vi "test FPGA DIO.vi"(8 "error in (no error)":errorcluster, 11 "TestCase in":refnum<class "cRIO System Tests.lvclass">) -> (0 "error out":errorcluster, 3 "TestCase out":refnum<class "cRIO System Tests.lvclass">)   [LabVIEW 2020, in "cRIO System Tests.lvclass"]
uses:
  cRIO System Tests.lvclass
  C:/Program Files (x86)/National Instruments/LabVIEW 2020/vi.lib/NI/VeriStand Custom Device Testing Tools/VeriStandTestCase/VeriStandTestCase.lvclass
  <vilib>/numeric/Random Number (Range) U64.vi
  <vilib>/numeric/sub_Random U32.vi
  <vilib>/addons/_JKI Toolkits/VI Tester/TestCase.llb/TestCase.lvclass
  <vilib>/NI/VeriStand Custom Device Testing Tools/VeriStandTestCase/VeriStandTestCase.lvclass
  C:/Program Files (x86)/National Instruments/LabVIEW 2020/vi.lib/addons/_JKI Toolkits/VI Tester/TestCase.llb/TestCase.lvclass
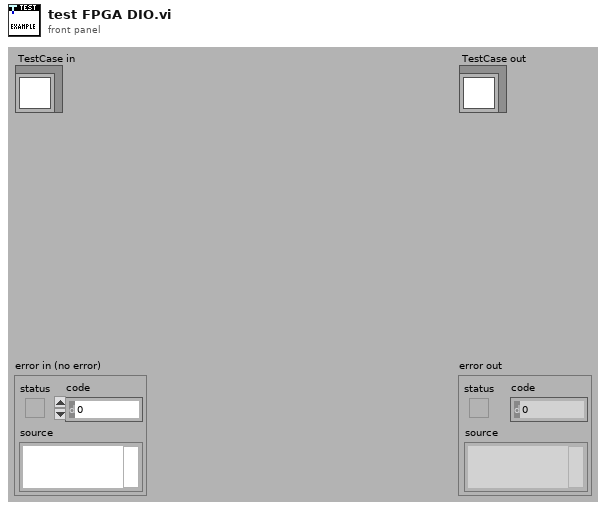
[diagram p1: front panel]
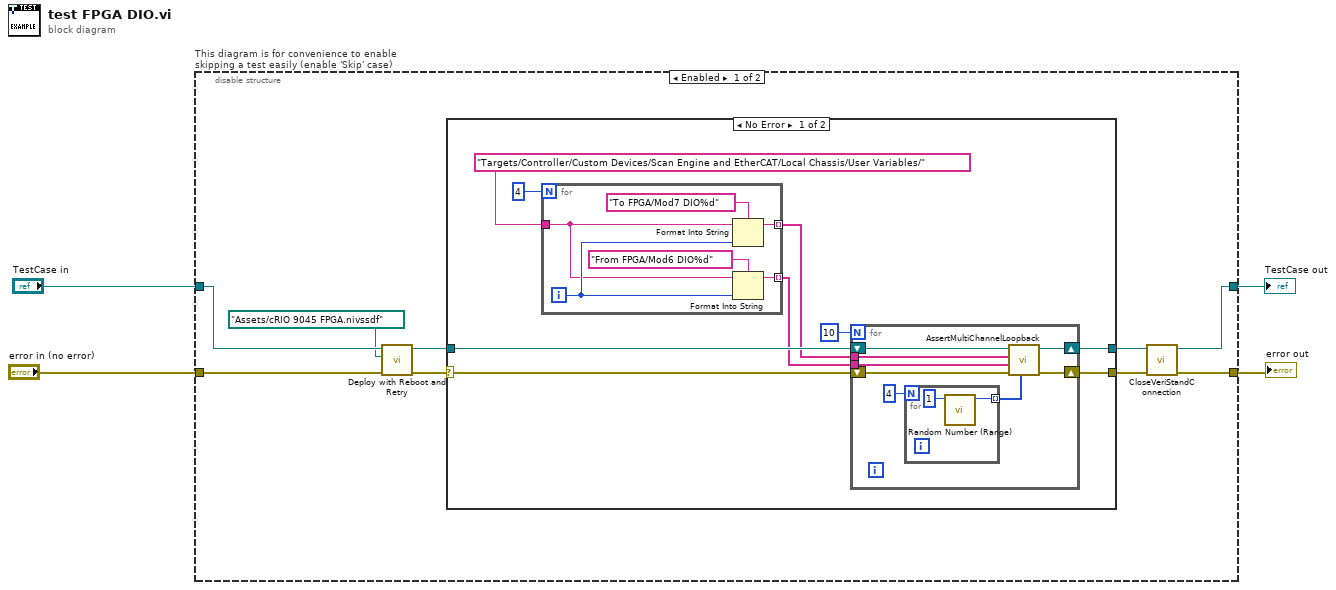
[diagram p0: block diagram]
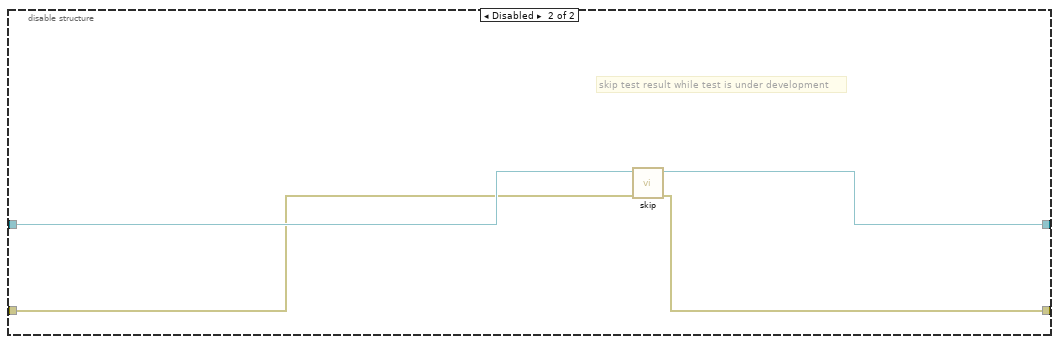
[diagram p3: hidden frame]
diagram:
  n1 = disable-structure "This diagram is for convenience to enable skipping a test easily (enable 'Skip' case)" shown="Enabled" {
    disable-tunnel: "TestCase in" -> [w10 w44]
    disable-tunnel: [w6 w42] -> w1
    disable-tunnel: [w8 w43] -> w3
    disable-tunnel: "error in (no error)" -> [w12 w41]
    frame Enabled {
      n2 = call "Deploy with Reboot and Retry.vi"("error in"=w12, "System Definition File"=path "Assets/cRIO 9045 FPGA.nivssdf", "VeriStand Test Case in"=w10) -> ("error out"=w13:errorcluster, "VeriStand Test Case out"=w11:refnum<class "cRIO System Tests.lvclass">)  [unwired: 7 in]
      n3 = case shown="No Error" w13 {
        selector: w13 -> [w18 w40]
        tunnel: [w17 w40] -> w9
        tunnel: [w19 w39] -> w7
        tunnel: w11 -> [w20 w39]
        frame No Error {
          n4 = for {
            N: 4 -> [_]
            tunnel: "Targets/Controller/Custom Devices/Scan Engine and EtherCAT/Local Chassis/User Variables/" -> [w35]
            tunnel: [w37] -> w16 mode=indexing
            tunnel: [w33] -> w15 mode=indexing
            i -> [w36]
            n5 = Format Into String(format string="To FPGA/Mod7 DIO%d", initial string=w35, w36) -> (resulting string=w37:string)  [unwired: 1 in, 1 out]
            n6 = Format Into String(format string="From FPGA/Mod6 DIO%d", initial string=w35, w36) -> (resulting string=w33:string)  [unwired: 1 in, 1 out]
          }
          n7 = for {
            N: 10 -> [_]
            tunnel: w16 -> [w26]
            tunnel: w15 -> [w25]
            shift-right: [w29] -> w19
            shift-left: w20 -> [w30]
            shift-right: [w27] -> w17
            shift-left: w18 -> [w28]
            n8 = for {
              N: 4 -> [_]
              tunnel: [w32] -> w23 mode=indexing
              n9 = call-poly <vilib>:"Random Number (Range).vi"("upper bound (100)"=u64 1) -> ("number"=w32:u64)  [unwired: 10 in]
            }
            n10 = call <vilib>:"AssertMultiChannelLoopback.vi"("Values"=w23, "error in (no error)"=w28, "Read Channels"=w25, "Write Channels"=w26, "VeriStand Test Case in"=w30) -> ("error out"=w27:errorcluster, "VeriStand Test Case out"=w29:refnum<class "cRIO System Tests.lvclass">)  [unwired: 5 in]
          }
        }
        frame Error {
        }
      }
      n11 = call-dynamic "CloseVeriStandConnection.vi"("error in (no error)"=w9, "VeriStand Test Case in"=w7) -> ("error out"=w8:errorcluster, "VeriStand Test Case out"=w6:refnum<class "cRIO System Tests.lvclass">)  [unwired: 8 in]
    }
    frame Disabled {
      # "skip test result while test is under development"
      n12 = call <vilib>:"skip.vi"("error in (no error)"=w41, "TestCase in"=w44) -> ("error out"=w43:errorcluster, "TestCase out"=w42:refnum<class "cRIO System Tests.lvclass">)  [unwired: 8 in]
    }
  }
  "error out" <- w3
  "TestCase out" <- w1
